vi "Sub_TermChannels.vi"(0 "Error In":errorcluster, 1 "Keithley In":refnum<visa-resource-name>) -> ()   [LabVIEW 2014]
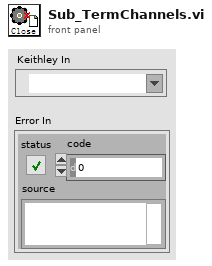
[diagram p1: front panel]
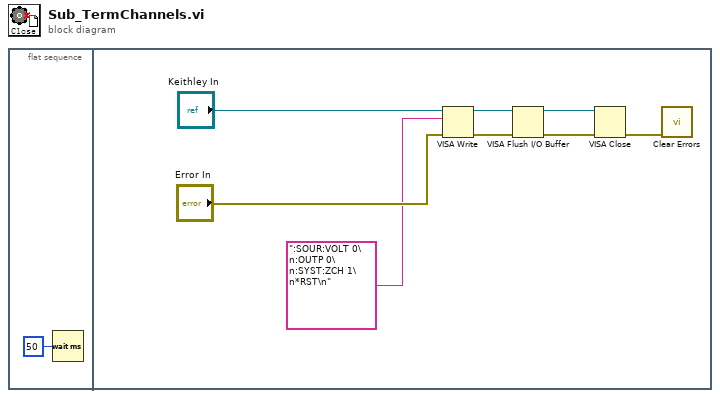
[diagram p0: block diagram]
diagram:
  n1 = flat-sequence {
    frame #0 {
      n2 = Wait (ms)(milliseconds to wait=u32 50) -> ()  [unwired: 1 out]
    }
    frame #1 {
      n3 = VISA Write(VISA resource name="Keithley In", write buffer=":SOUR:VOLT 0\n:OUTP 0\n:SYST:ZCH 1\n*RST\n", error in (no error)="Error In") -> (VISA resource name out=w6:refnum<visa-resource-name>, error out=w5:errorcluster)  [unwired: 1 out]
      n4 = VISA Flush I/O Buffer(VISA resource name=w6, error in (no error)=w5) -> (VISA resource name out=w4:refnum<visa-resource-name>, error out=w3:errorcluster)  [unwired: 1 in]
      n5 = VISA Close(VISA resource name=w4, error in (no error)=w3) -> (error out=w2:errorcluster)
      n6 = call <vilib>:"Clear Errors.vi"("error in (no error)"=w2) -> ()  [unwired: 5 in, 2 out]
    }
  }
